vi "FR GUI Connections.vi"() -> ()   [LabVIEW 2020]
doc: "GUI to show connection setup of the mesurement procedure used to estimate frequency response of the digitizer."
panel:
  in  "INRIM":bool
  in  "CMI":bool
  out "actual connection INRIM":picture
  out "actual connection CMI":picture
  in  "hide":bool
  # "Both setups are based on PTB\nmeasurement setup."
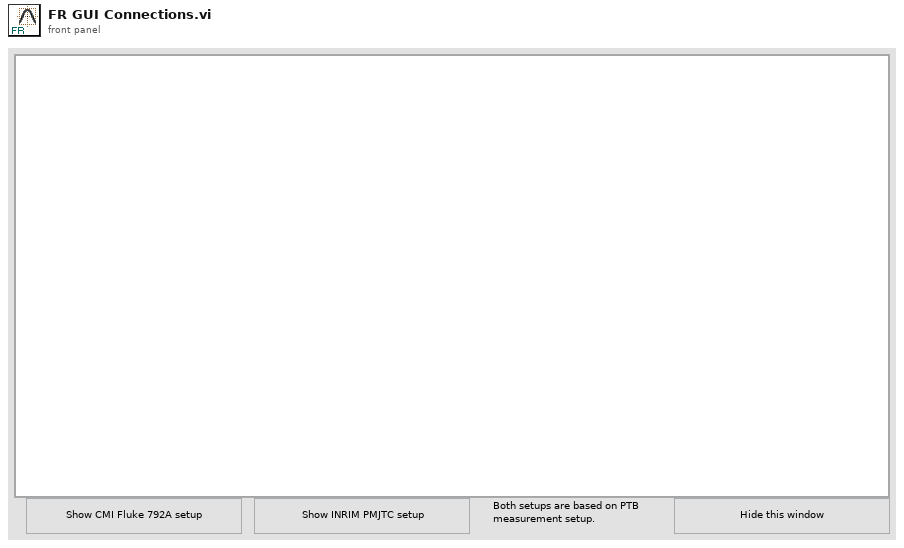
[diagram p1: front panel]
types:
  T1 = typedef "imagedata.ctl" = cluster{"image type":i32, "image depth":i32, "image":u8[], "mask":u8[], "colors":u32[], "Rectangle":cluster{"left":i16, "top":i16, "right":i16, "bottom":i16}}
  T2 = enum32{"Invalid", "Standard", "Closed", "Hidden", "Minimized", "Maximized"}
  T3 = typedef "LVRectTypeDef.ctl" = cluster{"Left":i16, "Top":i16, "Right":i16, "Bottom":i16}
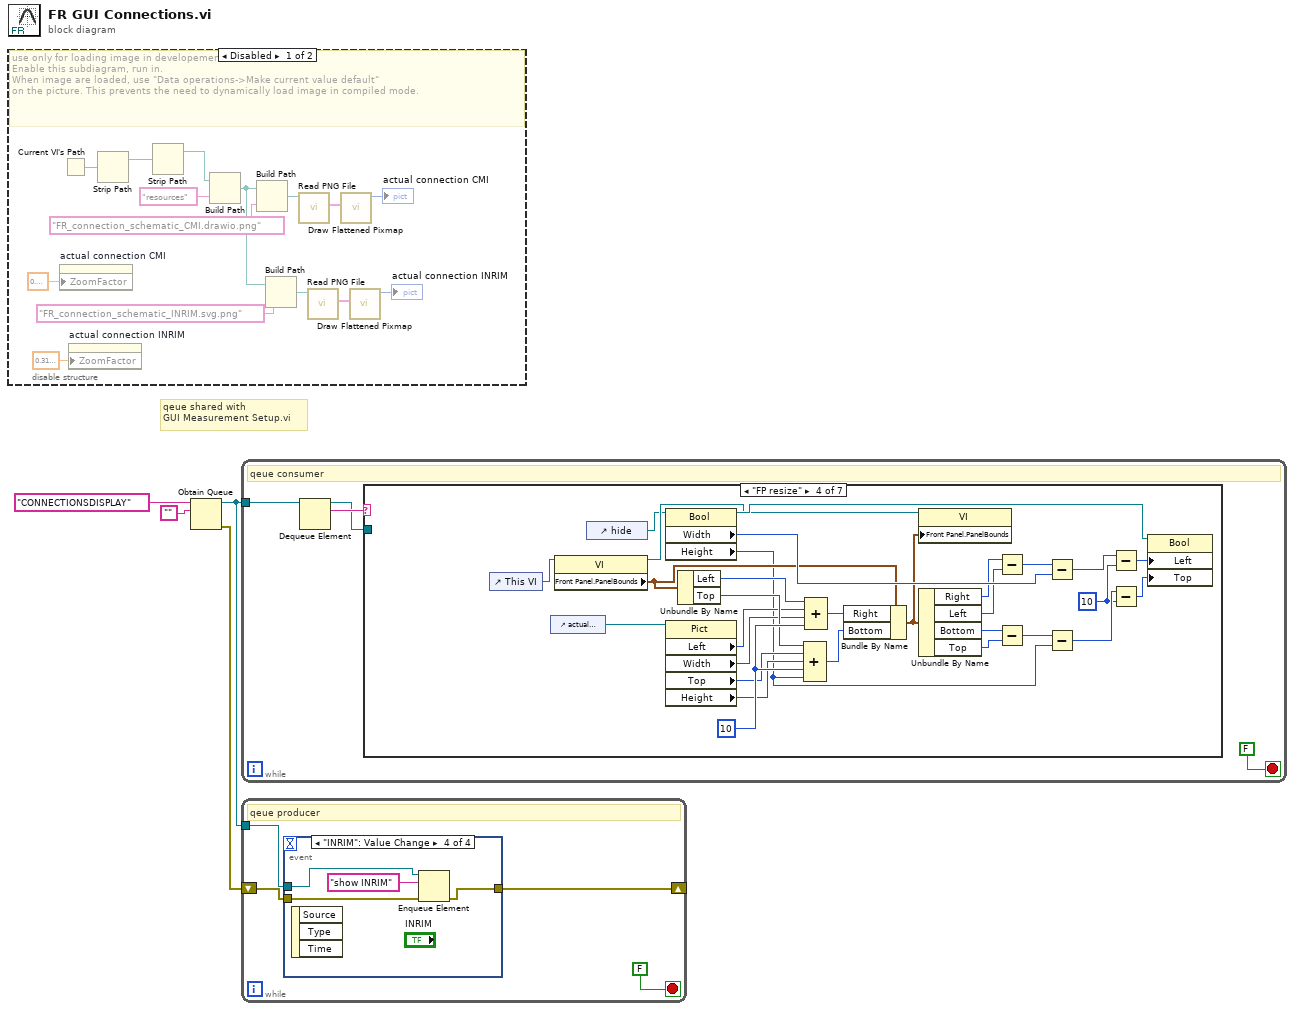
[diagram p0: block diagram]
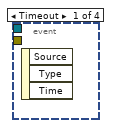
[diagram p2: hidden frame]
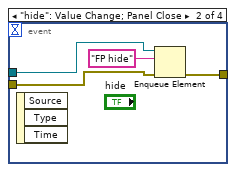
[diagram p3: hidden frame]
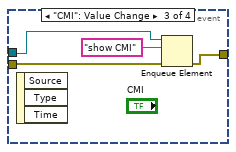
[diagram p4: hidden frame]
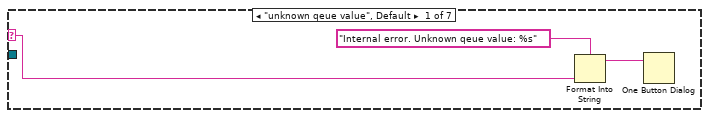
[diagram p5: hidden frame]
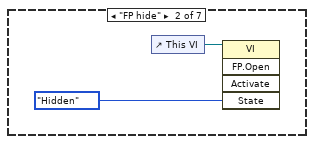
[diagram p6: hidden frame]
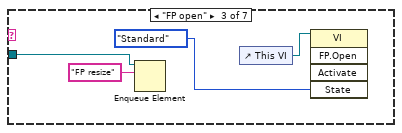
[diagram p7: hidden frame]
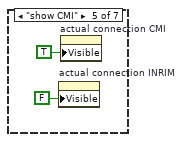
[diagram p8: hidden frame]
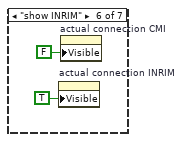
[diagram p9: hidden frame]
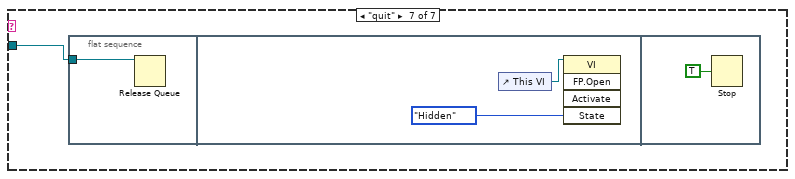
[diagram p10: hidden frame]
diagram:
  # "qeue shared with\nGUI Measurement Setup.vi"
  n1 = disable-structure shown="Disabled" {
    frame Disabled {
      # "use only for loading image in developement mode.\nEnable this subdiagram, run in.\nWhen image are loaded, use \"Data operations->Make current value default\" \non the picture. This prevents the need to dynamically load image in compiled mode."
      n2 = property on="actual connection CMI" class="Pict"("ZoomFactor"=sgl 0.4 ("Zoom Factor")) -> ()  [unwired: 2 in, 2 out]
      n3 = Current VI's Path() -> (path=w19:path)
      n4 = property on="actual connection INRIM" class="Pict"("ZoomFactor"=sgl 0.32 ("Zoom Factor")) -> ()  [unwired: 2 in, 2 out]
      n5 = Strip Path(path=w19) -> (stripped path=w18:path)  [unwired: 1 out]
      n6 = Strip Path(path=w18) -> (stripped path=w17:path)  [unwired: 1 out]
      n7 = Build Path(base path=w17, name or relative path="resources") -> (appended path=w6:path)
      n8 = Build Path(base path=w6, name or relative path="FR_connection_schematic_CMI.drawio.png") -> (appended path=w13:path)
      n9 = Build Path(base path=w6, name or relative path="FR_connection_schematic_INRIM.svg.png") -> (appended path=w9:path)
      n10 = call <vilib>:"Read PNG File.vi"("path to PNG file"=w13) -> ("image data"=w14:T1)  [unwired: 8 in, 2 out]
      n11 = call <vilib>:"Read PNG File.vi"("path to PNG file"=w9) -> ("image data"=w8:T1)  [unwired: 8 in, 2 out]
      n12 = call <vilib>:"Draw Flattened Pixmap.vi"("image data"=w14) -> ("new picture"=→"actual connection CMI":picture)  [unwired: 8 in]
      n13 = call <vilib>:"Draw Flattened Pixmap.vi"("image data"=w8) -> ("new picture"=→"actual connection INRIM":picture)  [unwired: 8 in]
    }
    frame Enabled {
    }
  }
  n14 = Obtain Queue(name (unnamed)="CONNECTIONSDISPLAY", element data type="" ("data (can be any type)")) -> (queue out=w1:refnum<queue>, error out=w2:errorcluster)  [unwired: 3 in, 1 out]
  n15 = while {
    tunnel: w1 -> [w22]
    stop <- FALSE stop-if-true
    # "qeue consumer"
    n16 = Dequeue Element(queue=w22) -> (queue out=w20:refnum<queue>, element=w21:string)  [unwired: 2 in, 2 out]
    n17 = case shown="\"FP resize\"" w21 {
      selector: w21 -> [w24 _ _ _ _ _ _]
      tunnel: w20 -> [_ _ w29 _ _ _ w66]
      frame "unknown qeue value", Default {
        n18 = Format Into String(format string="Internal error. Unknown qeue value: %s", w24) -> (resulting string=w26:string)  [unwired: 2 in, 1 out]
        n19 = One Button Dialog(message=w26) -> ()  [unwired: 1 in, 1 out]
      }
      frame "FP hide" {
        n20 = control-ref of="This VI"() -> (w27:refnum<vi>)
        n21 = invoke class="VI" method="FP.Open"(reference=w27, "State"=T2."Hidden") -> ()  [unwired: 3 in, 5 out]
      }
      frame "FP open" {
        n22 = Enqueue Element(queue=w29, element="FP resize") -> ()  [unwired: 2 in, 3 out]
        n23 = control-ref of="This VI"() -> (w31:refnum<vi>)
        n24 = invoke class="VI" method="FP.Open"(reference=w31, "State"=T2."Standard") -> ()  [unwired: 3 in, 5 out]
      }
      frame "FP resize" {
        w42 = u32 10 ("value")
        w47 = u32 10 ("y")
        n25 = control-ref of="This VI"() -> (w49:refnum<vi>)
        n26 = control-ref of="actual connection CMI"() -> (w33:refnum<vi>)
        n27 = property class="VI"(reference=w49) -> (reference out=w48:refnum<vi>, "Front Panel.PanelBounds"=w45:T3)  [unwired: 1 in, 1 out]
        n28 = control-ref of="hide"() -> (w34:refnum<vi>)
        n29 = property class="Bool"(reference=w34) -> (reference out=w61:refnum<vi>, "Width"=w60:u32, "Height"=w36:u32)  [unwired: 1 in, 1 out]
        n30 = property class="Pict"(reference=w33) -> ("Left"=w38:i32, "Width"=w39:u32, "Top"=w37:i32, "Height"=w41:u32)  [unwired: 1 in, 2 out]
        n31 = Unbundle By Name(w45) -> ("Left"=w46:i16, "Top"=w40:i16)
        n32 = Compound Arithmetic op=ADD(w40, w37, w41, w42, w36) -> (w43:u32)
        n33 = Compound Arithmetic op=ADD(w46, w38, w39, w42) -> (w44:u32)
        n34 = Bundle By Name(cluster=w45, "Right"=w44, "Bottom"=w43) -> (w35:T3)
        n35 = property class="VI"(reference=w48, "Front Panel.PanelBounds"=w35) -> ()  [unwired: 1 in, 2 out]
        n36 = Unbundle By Name(w35) -> ("Right"=w55:i16, "Left"=w54:i16, "Bottom"=w58:i16, "Top"=w56:i16)
        n37 = Subtract(x=w55, y=w54) -> (x-y=w59:i16)
        n38 = Subtract(x=w58, y=w56) -> (x-y=w57:i16)
        n39 = Subtract(x=w59, y=w60) -> (x-y=w53:u32)
        n40 = Subtract(x=w57, y=w36) -> (x-y=w52:u32)
        n41 = Subtract(x=w53, y=w47) -> (x-y=w51:u32)
        n42 = Subtract(x=w52, y=w47) -> (x-y=w50:u32)
        n43 = property class="Bool"(reference=w61, "Left"=w51, "Top"=w50) -> ()  [unwired: 1 in, 2 out]
      }
      frame "show CMI" {
        n44 = property on="actual connection INRIM" class="Pict"("Visible"=FALSE) -> ()  [unwired: 2 in, 2 out]
        n45 = property on="actual connection CMI" class="Pict"("Visible"=TRUE) -> ()  [unwired: 2 in, 2 out]
      }
      frame "show INRIM" {
        n46 = property on="actual connection INRIM" class="Pict"("Visible"=TRUE) -> ()  [unwired: 2 in, 2 out]
        n47 = property on="actual connection CMI" class="Pict"("Visible"=FALSE) -> ()  [unwired: 2 in, 2 out]
      }
      frame "quit" {
        n48 = flat-sequence {
          tunnel: w66 -> [w67]
          frame #0 {
            n49 = Release Queue(queue=w67) -> ()  [unwired: 2 in, 3 out]
          }
          frame #1 {
            n50 = control-ref of="This VI"() -> (w68:refnum<vi>)
            n51 = invoke class="VI" method="FP.Open"(reference=w68, "State"=T2."Hidden") -> ()  [unwired: 3 in, 5 out]
          }
          frame #2 {
            n52 = Stop(stop? (T)=TRUE) -> ()
          }
        }
      }
    }
  }
  n53 = while {
    shift-right: [w73] -> _
    shift-left: w2 -> [w74]
    tunnel: w1 -> [w72]
    stop <- FALSE stop-if-true
    # "qeue producer"
    n54 = event shown="[3] \"INRIM\": Value Change" {
      selector: _ -> [_ _ _ _]
      dyn-events: _ -> [_ _ _ _]
      timeout: _ -> [_ _ _ _]
      tunnel: w74 -> [_ w77 w81 w85]
      tunnel: [_ w76 w79 w84] -> w73
      tunnel: w72 -> [_ w75 w80 w83]
      event Timeout {
        n55 = event-data() -> ()  [unwired: 1 in, 3 out]
      }
      event "hide": Value Change; Panel Close {
        n56 = event-data() -> ()  [unwired: 1 in, 3 out]
        n57 = Enqueue Element(queue=w75, element="FP hide", error in (no error)=w77) -> (error out=w76:errorcluster)  [unwired: 1 in, 2 out]
      }
      event "CMI": Value Change {
        n58 = event-data() -> ()  [unwired: 1 in, 3 out]
        n59 = Enqueue Element(queue=w80, element="show CMI", error in (no error)=w81) -> (error out=w79:errorcluster)  [unwired: 1 in, 2 out]
      }
      event "INRIM": Value Change {
        n60 = event-data() -> ()  [unwired: 1 in, 3 out]
        n61 = Enqueue Element(queue=w83, element="show INRIM", error in (no error)=w85) -> (error out=w84:errorcluster)  [unwired: 1 in, 2 out]
      }
    }
  }
